vi "SetBuvVoltage (SubVI).vi"(0 "connection ID in":refnum<k5>, 3 "BuvV2set":dbl, 5 "error in":errorcluster) -> (14 "connection ID out":refnum<k5>, 19 "error out":errorcluster)   [LabVIEW 2013]
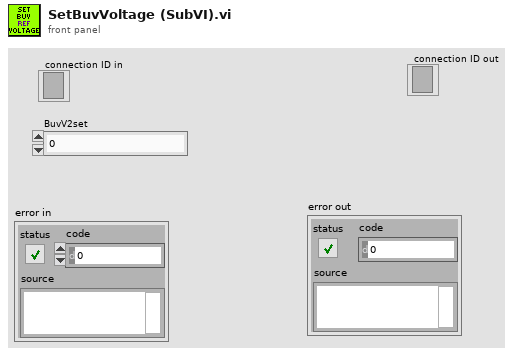
[diagram p1: front panel]
types:
  T1 = enum16{"Standard", "Buffered", "CRLF", "Immediate"}
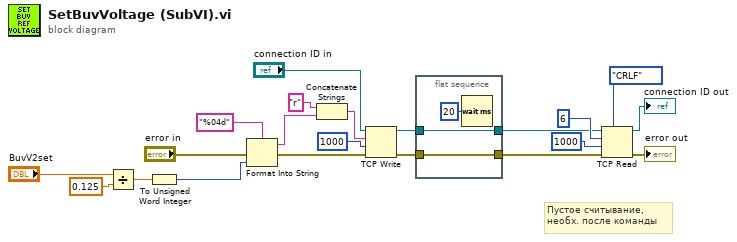
[diagram p0: block diagram]
diagram:
  # "Пустое считывание,\nнеобх. после команды"
  n1 = Divide(x="BuvV2set", y=0.125) -> (x/y=w14:dbl)
  n2 = To Unsigned Word Integer(number=w14) -> (unsigned 16bit integer=w1:u16)
  n3 = Format Into String(format string="%04d", error in="error in", w1) -> (resulting string=w18:string, error out=w11:errorcluster)  [unwired: 1 in]
  n4 = Concatenate Strings("r" ("data in"), w18) -> (w19:string)
  n5 = TCP Write(connection ID="connection ID in", data in=w19, error in (no error)=w11, 9:1000 ("timeout ms (25000)")) -> (connection ID out=w16:refnum<k5>, error out=w15:errorcluster)  [unwired: 1 out]
  n6 = flat-sequence {
    tunnel: [w24] -> w2
    tunnel: w16 -> [w24]
    tunnel: [w23] -> w3
    tunnel: w15 -> [w23]
    frame #0 {
      n7 = Wait (ms)(milliseconds to wait=u32 20) -> ()  [unwired: 1 out]
    }
  }
  n8 = TCP Read(connection ID=w2, bytes to read=6, error in (no error)=w3, 7:T1."CRLF" ("mode (standard)"), 9:1000 ("timeout ms (25000)")) -> (connection ID out=→"connection ID out":refnum<k5>, error out=→"error out":errorcluster)  [unwired: 1 out]
